vi "1-shift.vi"(2 "this":i32, 3 "button":i32) -> (0 "shift":bool, 1 "next state":i32)   [LabVIEW 2017]
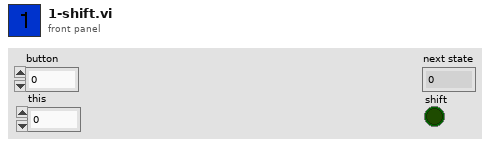
[diagram p1: front panel]
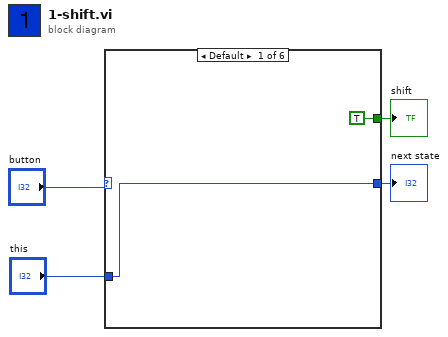
[diagram p0: block diagram]
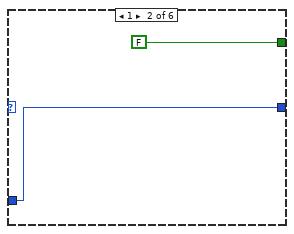
[diagram p2: hidden frame]
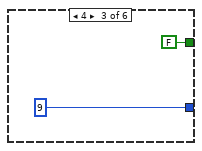
[diagram p3: hidden frame]
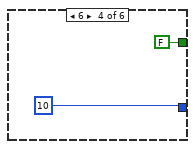
[diagram p4: hidden frame]
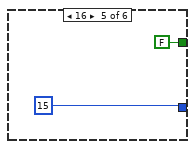
[diagram p5: hidden frame]
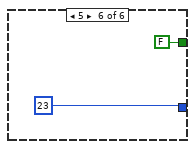
[diagram p6: hidden frame]
diagram:
  n1 = case shown="Default" "button" {
    tunnel: [w6 w8 9 10 15 23] -> w3
    tunnel: "this" -> [w6 w8 _ _ _ _]
    tunnel: [TRUE FALSE FALSE FALSE FALSE FALSE] -> w1
    frame Default {
    }
    frame 1 {
    }
    frame 4 {
    }
    frame 6 {
    }
    frame 16 {
    }
    frame 5 {
    }
  }
  "next state" <- w3
  "shift" <- w1
